vi "ParseXBee.vi"(2 "XBee String":string) -> (0 "Bump 1":bool, 1 "Bump 2":bool, 3 "IR 1":dbl, 4 "IR 2":dbl, 5 "Red":dbl, 6 "Blue":dbl, 7 "Green":dbl, 8 "X":dbl, 9 "Y":dbl, 10 "Z":dbl)   [LabVIEW 2012]
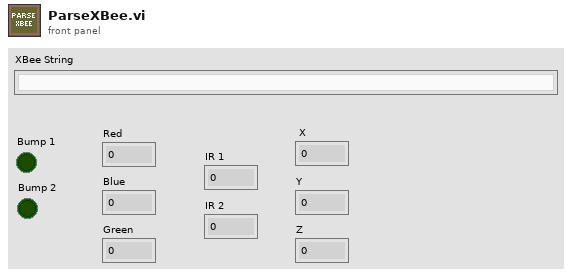
[diagram p1: front panel]
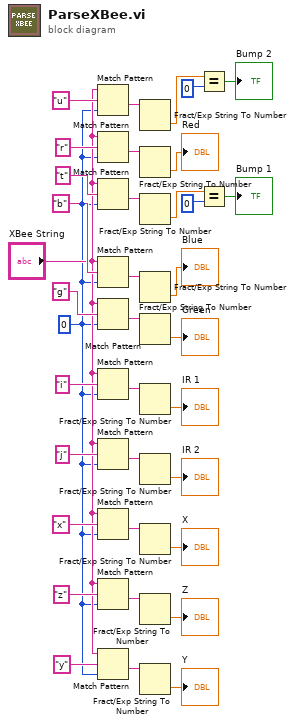
[diagram p0: block diagram]
diagram:
  w4 = 0 ("offset (0)")
  n1 = Match Pattern(string="XBee String", regular expression="u", offset (0)=w4) -> (after substring=w23:string)  [unwired: 3 out]
  n2 = Match Pattern(string="XBee String", regular expression="r", offset (0)=w4) -> (after substring=w30:string)  [unwired: 3 out]
  n3 = Match Pattern(string="XBee String", regular expression="t", offset (0)=w4) -> (after substring=w27:string)  [unwired: 3 out]
  n4 = Match Pattern(string="XBee String", regular expression="b", offset (0)=w4) -> (after substring=w28:string)  [unwired: 3 out]
  n5 = Match Pattern(string="XBee String", regular expression="g", offset (0)=w4) -> (after substring=w29:string)  [unwired: 3 out]
  n6 = Match Pattern(string="XBee String", regular expression="i", offset (0)=w4) -> (after substring=w31:string)  [unwired: 3 out]
  n7 = Match Pattern(string="XBee String", regular expression="j", offset (0)=w4) -> (after substring=w25:string)  [unwired: 3 out]
  n8 = Match Pattern(string="XBee String", regular expression="x", offset (0)=w4) -> (after substring=w10:string)  [unwired: 3 out]
  n9 = Match Pattern(string="XBee String", regular expression="z", offset (0)=w4) -> (after substring=w6:string)  [unwired: 3 out]
  n10 = Match Pattern(string="XBee String", regular expression="y", offset (0)=w4) -> (after substring=w8:string)  [unwired: 3 out]
  n11 = Fract/Exp String To Number(string=w23) -> (number=w17:dbl)  [unwired: 3 in, 1 out]
  n12 = Fract/Exp String To Number(string=w30) -> (number=→"Red":dbl)  [unwired: 3 in, 1 out]
  n13 = Fract/Exp String To Number(string=w27) -> (number=w18:dbl)  [unwired: 3 in, 1 out]
  n14 = Fract/Exp String To Number(string=w28) -> (number=→"Blue":dbl)  [unwired: 3 in, 1 out]
  n15 = Fract/Exp String To Number(string=w29) -> (number=→"Green":dbl)  [unwired: 3 in, 1 out]
  n16 = Fract/Exp String To Number(string=w31) -> (number=→"IR 1":dbl)  [unwired: 3 in, 1 out]
  n17 = Fract/Exp String To Number(string=w25) -> (number=→"IR 2":dbl)  [unwired: 3 in, 1 out]
  n18 = Fract/Exp String To Number(string=w10) -> (number=→"X":dbl)  [unwired: 3 in, 1 out]
  n19 = Fract/Exp String To Number(string=w6) -> (number=→"Z":dbl)  [unwired: 3 in, 1 out]
  n20 = Fract/Exp String To Number(string=w8) -> (number=→"Y":dbl)  [unwired: 3 in, 1 out]
  n21 = Equal?(x=w17, y=0) -> (x = y?=→"Bump 2":bool)
  n22 = Equal?(x=w18, y=0) -> (x = y?=→"Bump 1":bool)
